vi "oax_Generate Simulated Vibration and Tach Signal.vi"(5 "reset?":bool=TRUE, 7 "fs":dbl, 9 "order info":T1(array[cluster]) {"envelop config"."low limit" format="%.2f"; "envelop config"."high limit" format="%.2f"; "envelop config"."f" format="%.2f"; "AM selection" items=["None", "Sine", "Triangle"]}, 10 "time period":dbl[](array[numeric]), 11 "speed":dbl[](array[numeric])) -> (2 "Tach Signal":waveform(dbl), 3 "Vibration Signal":waveform(dbl))   [LabVIEW 2017]
panel:
  out "Waveform Graph":waveform(dbl)[](graph)
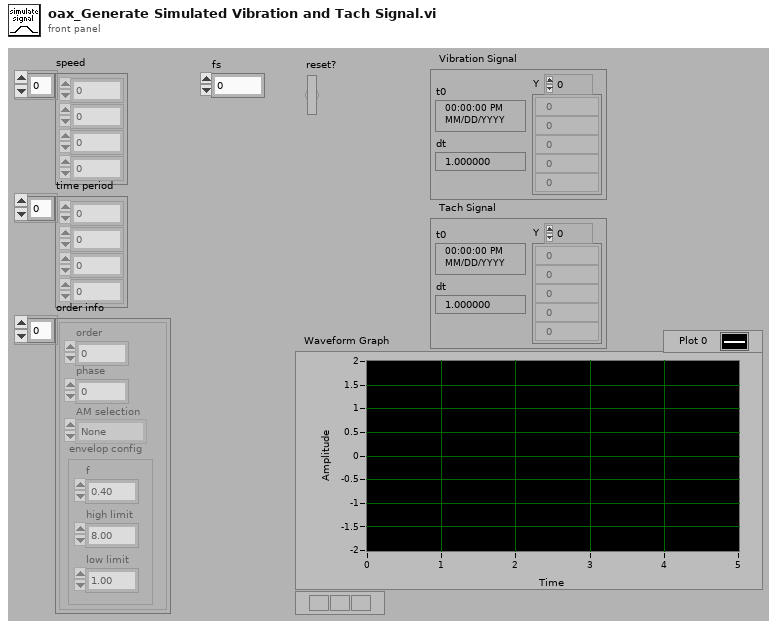
[diagram p1: front panel]
types:
  T1 = cluster{"order":dbl, "phase":dbl, "AM selection":u16, "envelop config":cluster{"f":dbl, "high limit":dbl, "low limit":dbl}}[]
  T2 = cluster{"f":dbl, "high limit":dbl, "low limit":dbl}
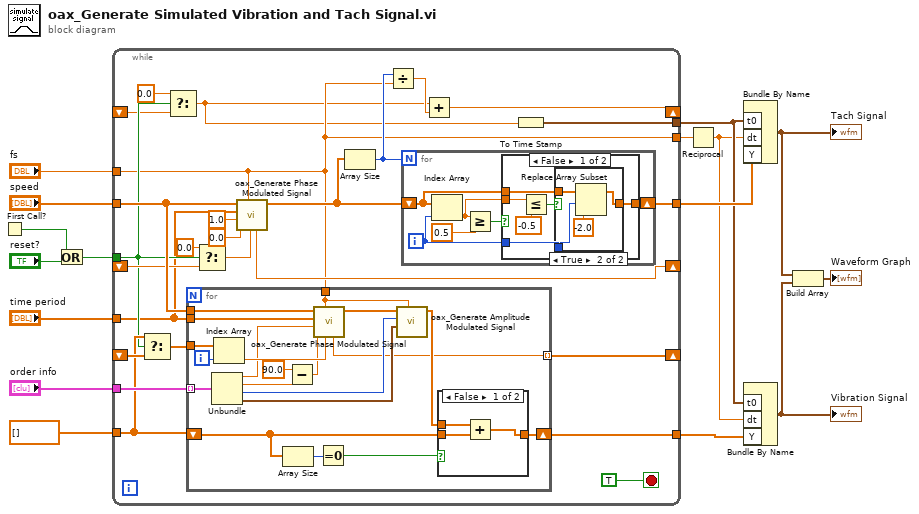
[diagram p0: block diagram]
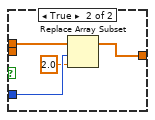
[diagram p3: hidden frame]
diagram:
  n1 = First Call?() -> (First Call?: T/F=w8:bool)
  n2 = Or(x=w8, y="reset?") -> (x .or. y?=w6:bool)
  n3 = while {
    tunnel: [w27] -> w16
    tunnel: "order info" -> [w41]
    tunnel: "fs" -> [w19]
    tunnel: "speed" -> [w40]
    tunnel: "time period" -> [w24]
    tunnel: dbl[] [] ("time period 2") -> [w29]
    tunnel: [w28] -> w10
    tunnel: [w19] -> w5
    tunnel: [w39] -> w9
    shift-right: [w37] -> _
    shift-left: _ -> [w35]
    tunnel: w6 -> [w26]
    shift-right: [w32] -> _
    shift-left: _ -> [w31]
    shift-right: [w22] -> _
    shift-left: _ -> [w23]
    stop <- TRUE stop-if-true
    n4 = Select(t=w29, s=w26, f=w31) -> (s? t:f=w30:dbl[])
    n5 = Select(t=0.0, s=w26, f=w23) -> (s? t:f=w17:dbl)
    n6 = for {
      tunnel: w41 -> [w83] mode=indexing
      tunnel: w19 -> [w72]
      tunnel: w40 -> [w82]
      tunnel: w24 -> [w81]
      shift-right: [w74] -> w28
      shift-left: w29 -> [w77]
      tunnel: [w71] -> w32 mode=indexing
      tunnel: w30 -> [w70]
      i -> [w69]
      n7 = Unbundle(w83) -> ("order"=w67:dbl, "phase"=w66:dbl, "AM selection"=w79:u16, "envelop config"=w78:T2)
      n8 = Index Array(array=w70, index=w69) -> (element=w68:dbl)
      n9 = Array Size(array=w77) -> (size(s)=w76:i32)
      n10 = Subtract(x=90.0, y=w66) -> (x-y=w64:dbl)
      n11 = call <vilib>:"oax_Generate Phase Modulated Signal.vi"("init phase"=w68, "fs"=w72, "phase"=w64, "order"=w67, "time period"=w81, "speed"=w82) -> ("y"=w80:dbl[], "final phase"=w71:dbl)  [unwired: 4 in]
      n12 = Equal To 0?(x=w76) -> (x = 0?=w75:bool)
      n13 = call <vilib>:"oax_Generate Amplitude Modulated Signal.vi"("fs"=w72, "envelop config"=w78, "AM selection"=w79, "x"=w80) -> ("AM modulated signal"=w73:dbl[])  [unwired: 7 in]
      n14 = case shown="False" w75 {
        tunnel: w77 -> [w85 _]
        tunnel: [w84 w87] -> w74
        tunnel: w73 -> [w86 w87]
        frame False {
          n15 = Add(x=w86, y=w85) -> (x+y=w84:dbl[])
        }
        frame True {
        }
      }
    }
    n16 = Select(t=0.0 ("phase"), s=w26, f=w35) -> (s? t:f=w34:dbl)
    n17 = call <vilib>:"oax_Generate Phase Modulated Signal.vi"("init phase"=w34, "fs"=w19, "phase"=0.0, "order"=1.0, "time period"=w24, "speed"=w40) -> ("y"=w21:dbl[], "final phase"=w37:dbl)  [unwired: 4 in]
    n18 = Array Size(array=w21) -> (size(s)=w20:i32)
    n19 = Divide(x=w20, y=w19) -> (x/y=w18:dbl)
    n20 = for {
      N: w20 -> [_]
      shift-right: [w44] -> w27
      shift-left: w21 -> [w46]
      i -> [w45]
      n21 = Index Array(array=w46, index=w45) -> (element=w43:dbl)
      n22 = Greater Or Equal?(x=w43, y=0.5) -> (x >= y?=w47:bool)
      n23 = case shown="False" w47 {
        tunnel: w46 -> [w50 w63]
        tunnel: w45 -> [w49 w62]
        tunnel: [w51 w60] -> w44
        tunnel: w43 -> [w53 _]
        frame False {
          n24 = Less Or Equal?(x=w53, y=-0.5) -> (x <= y?=w52:bool)
          n25 = case shown="True" w52 {
            tunnel: [w55 w58] -> w51
            tunnel: w50 -> [w55 w59]
            tunnel: w49 -> [_ w57]
            frame False {
            }
            frame True {
              n26 = Replace Array Subset(array=w59, new element=-2.0 ("y"), index=w57) -> (w58:dbl[])
            }
          }
        }
        frame True {
          n27 = Replace Array Subset(array=w63, new element=2.0 ("new element/subarray"), index=w62) -> (w60:dbl[])
        }
      }
    }
    n28 = Add(x=w17, y=w18) -> (x+y=w22:dbl)
    n29 = To Time Stamp(1:w17) -> (0:w39:timestamp)
  }
  n30 = Reciprocal(x=w5) -> (1/x=w4:dbl)
  n31 = Bundle By Name("t0"=w9, "dt"=w4, "Y"=w16) -> (w1:waveform(dbl))  [unwired: 1 in]
  "Tach Signal" <- w1
  n32 = Bundle By Name("t0"=w9, "dt"=w4, "Y"=w10) -> (w2:waveform(dbl))  [unwired: 1 in]
  "Vibration Signal" <- w2
  n33 = Build Array(w1, w2) -> (→"Waveform Graph":waveform(dbl)[])
